vi "Read Key (DBL).vi"(7 "Section Name":string, 8 "error in (no error)":errorcluster, 9 "Default":dbl, 10 "Key Name":string, 11 "Config in":T1) -> (0 "error out":errorcluster, 1 "Value":dbl, 2 "Key Found?":bool, 3 "Config out":T1)   [LabVIEW 2022 SP3, in "LabVIEW-Config.lvlib"]
uses:
  LabVIEW-Config.lvlib
  Config.ctl
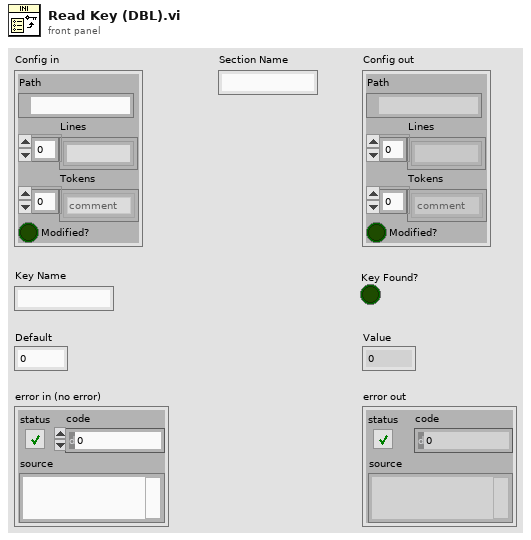
[diagram p1: front panel]
types:
  T1 = typedef "LabVIEW-Config.lvlib/Config.ctl" = cluster{"Path":path, "Lines":string[], "Tokens":enum8{"comment", "section", "key"}[], "Modified?":bool}
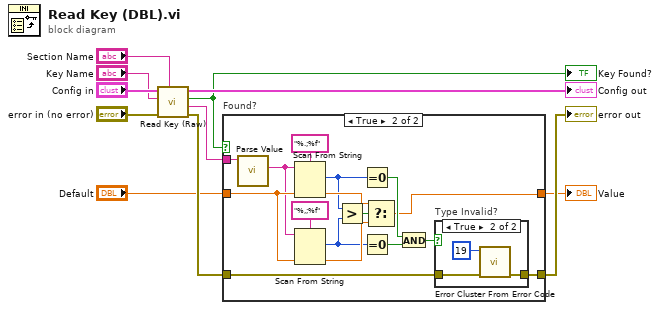
[diagram p0: block diagram]
diagram:
  n1 = call "Read Key (Raw).vi"("Section Name"="Section Name", "error in (no error)"="error in (no error)", "Key Name"="Key Name", "Config in"="Config in") -> ("error out"=w4:errorcluster, "Content"=w6:string, "Key Found?"=w3:bool, "Config out"=→"Config out":T1)  [unwired: 4 in]
  "Key Found?" <- w3
  n2 = case "Found?" shown="True" w3 {
    tunnel: w6 -> [_ w29]
    tunnel: [w13 w14] -> w1
    tunnel: "Default" -> [w13 w17]
    tunnel: [w12 w28] -> w5
    tunnel: w4 -> [w12 w27]
    frame False {
    }
    frame True {
      n3 = call "Parse Value.vi"("Value"=w29) -> ("Value (Comment Removed)"=w16:string)  [unwired: 9 in, 1 out]
      n4 = Scan From String(format string="%.;%f" ("Format String"), input string=w16, default 1=w17) -> (offset past scan=w21:u32, output 1=w23:dbl)  [unwired: 2 in, 2 out]
      n5 = Scan From String(format string="%,;%f" ("Format String"), input string=w16, default 1=w17) -> (offset past scan=w20:u32, output 1=w22:dbl)  [unwired: 2 in, 2 out]
      n6 = Greater?(x=w21, y=w20) -> (0:w24:bool)
      n7 = Equal To 0?(x=w21) -> (x = 0?=w18:bool)
      n8 = Equal To 0?(x=w20) -> (x = 0?=w19:bool)
      n9 = Select(t=w23, s=w24, f=w22) -> (s? t:f=w14:dbl)
      n10 = And(x=w18, y=w19) -> (x .and. y?=w15:bool)
      n11 = case "Type Invalid?" shown="True" w15 {
        tunnel: w27 -> [w30 w32]
        tunnel: [w30 w31] -> w28
        frame False {
        }
        frame True {
          n12 = call <vilib>:"Error Cluster From Error Code.vi"("error in (no error)"=w32, "error code (0)"=19 ("Type invalid")) -> ("error out"=w31:errorcluster)  [unwired: 7 in]
        }
      }
    }
  }
  "error out" <- w5
  "Value" <- w1
